vi "ActiveConfigWindow.vi"   [LabVIEW 2015, in "ConfigHelper.lvlib"]
uses:
  ConfigHelper.lvlib
  ConfigWindow.vi
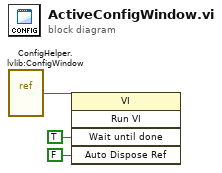
[diagram p0: block diagram]
diagram:
  n1 = vi-ref "ConfigHelper.lvlib:ConfigWindow.vi"() -> (w1:refnum<vi>)
  n2 = invoke class="VI" method="Run VI"(reference=w1, "Wait until done"=TRUE ("Wait Until Done"), "Auto Dispose Ref"=FALSE ("Auto Dispose Reference")) -> ()  [unwired: 2 in, 5 out]
